vi "Stack_Init.vi"(0 "object in":refnum<class "Stack.lvclass">, 11 "Error In":errorcluster) -> (4 "object out":refnum<class "Stack.lvclass">, 15 "Error Out":errorcluster)   [LabVIEW 2024, in "Stack.lvclass"]
uses:
  Stack.lvclass
  Stack.lvclass/Stack.ctl
panel:
  # "Connector Pane"
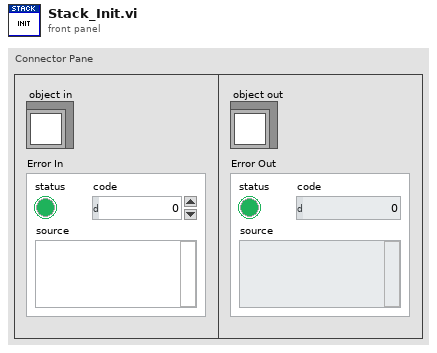
[diagram p1: front panel]
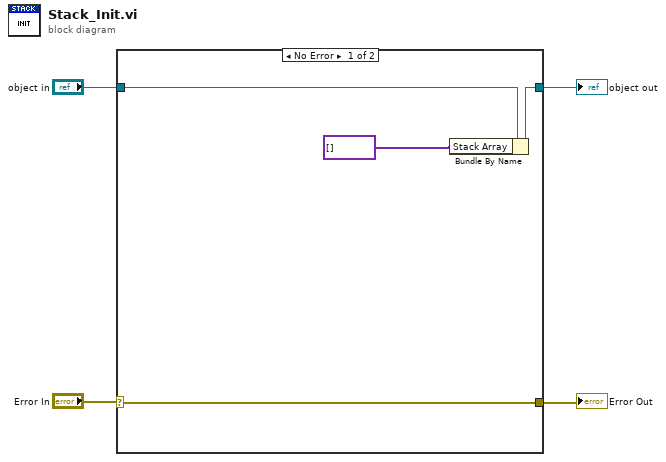
[diagram p0: block diagram]
diagram:
  n1 = case shown="No Error" "Error In" {
    selector: "Error In" -> [w6 w9]
    tunnel: "object in" -> [w8 w10]
    tunnel: [w7 w10] -> w3
    tunnel: [w6 w9] -> w1
    frame No Error {
      n2 = Bundle By Name(cluster=w8, "Stack Array"=variant[] []) -> (w7:refnum<class "Stack.lvclass">)
    }
    frame Error {
    }
  }
  "object out" <- w3
  "Error Out" <- w1
